vi "main0.1.vi"() -> ()   [LabVIEW 2025]
uses:
  STATES_MACHINE.ctl
  <vilib>/Utility/file.llb/Write Delimited Spreadsheet (DBL).vi
panel:
  out "array":dbl[][](array[numeric]) format="%#_5g"
  out "Enum":T1
  in  "Stop Generale":bool
  in  "Aggiungi caso":bool
  out "Outlet":dbl
  out "Secondary":dbl
  out "Primary":dbl
  out "Waveform Graph":dynamicdata(graph)
  in  "Altro test":bool
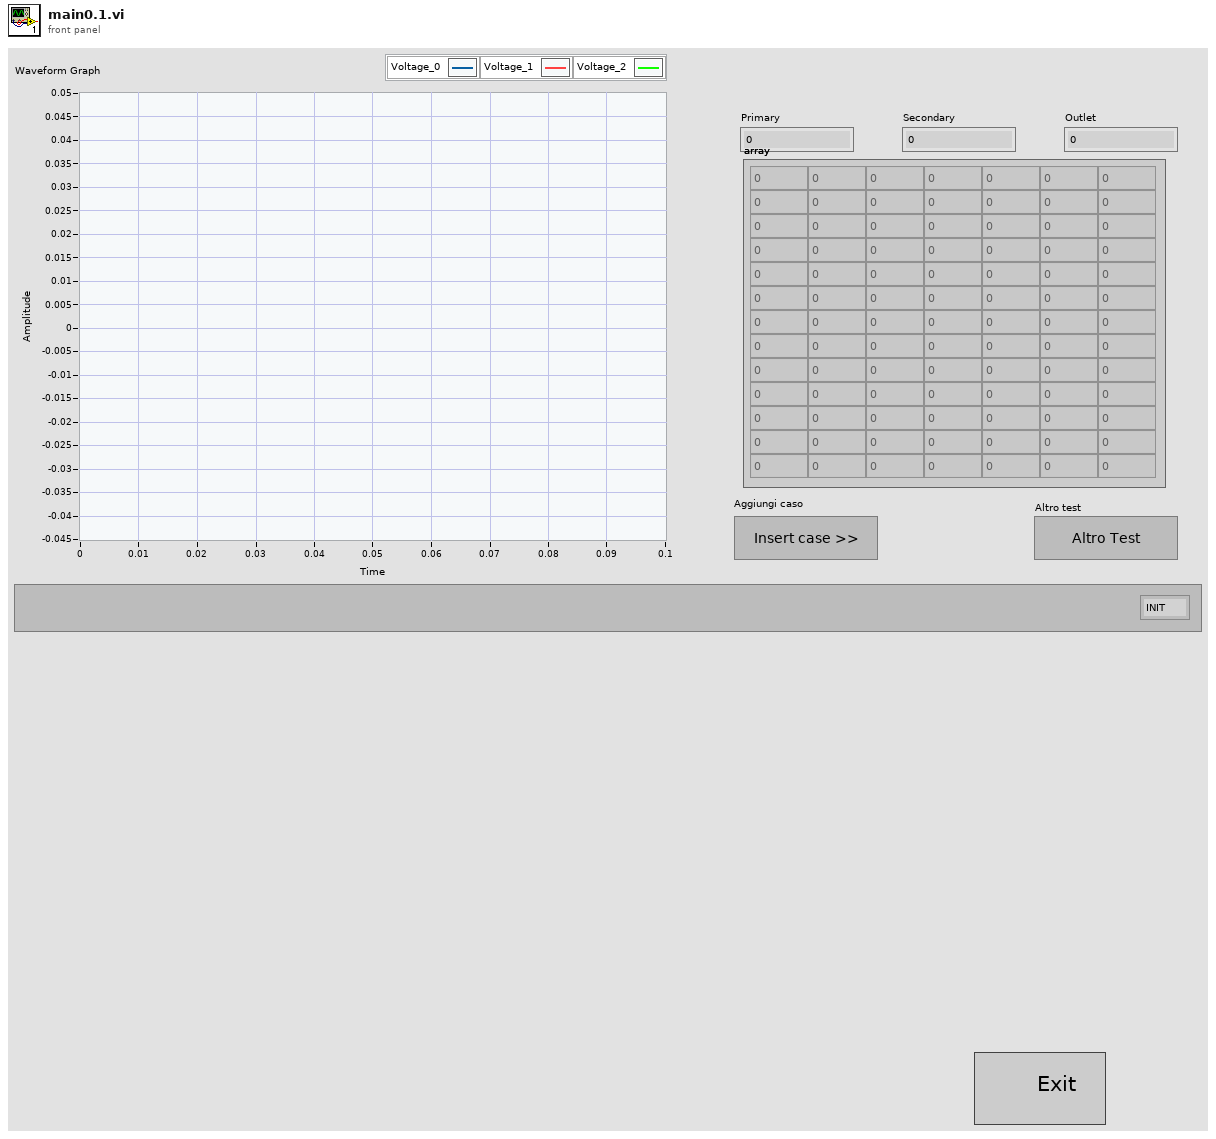
[diagram p1: front panel]
types:
  T1 = typedef "STATES_MACHINE.ctl" = enum16{"INIT", "TEST", "WRITE_RESULT", "CLOSE"}
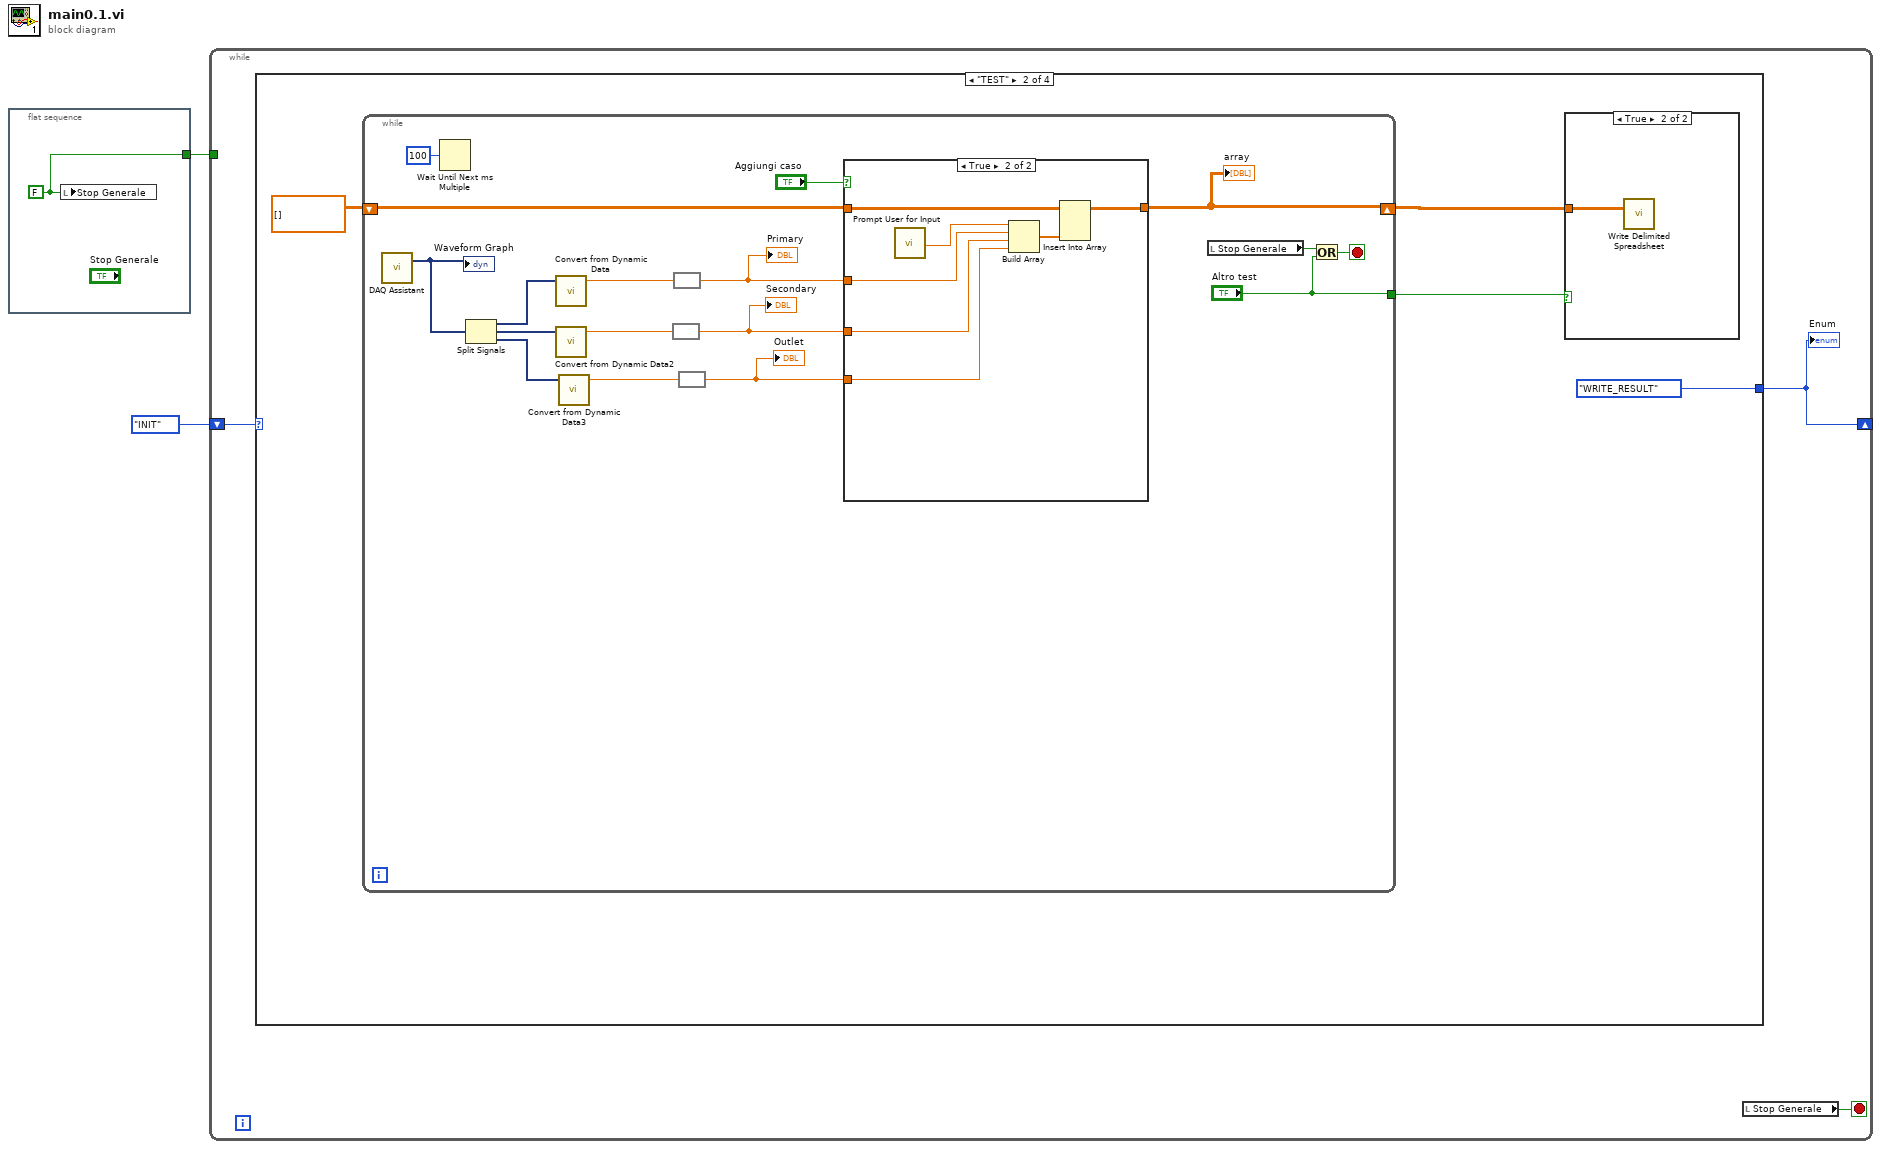
[diagram p0: block diagram]
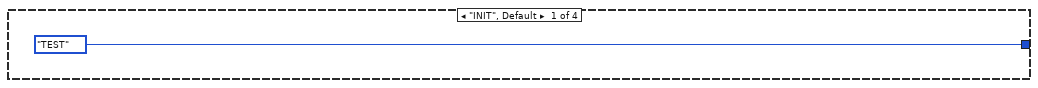
[diagram p2: hidden frame]
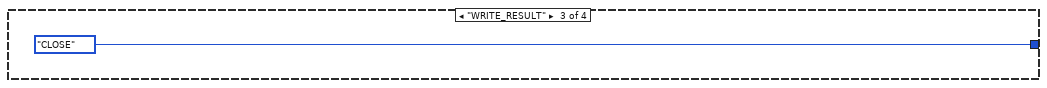
[diagram p5: hidden frame]
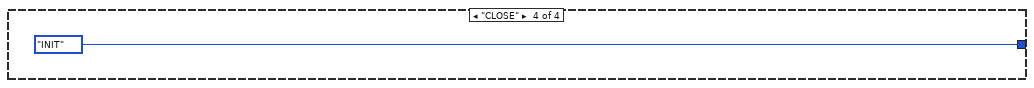
[diagram p6: hidden frame]
diagram:
  n1 = flat-sequence {
    tunnel: [w3] -> w1
    frame #0 {
      w3 = FALSE ("Stop Button 2")
      n2 = local write "Stop Generale"(w3) -> ()
    }
  }
  n3 = while {
    shift-right: [w5] -> _
    shift-left: STATES_MACHINE."INIT" ("Enum") -> [w6]
    tunnel: w1 -> [_]
    stop <- w4 stop-if-true
    n4 = case shown="\"TEST\"" w6 {
      tunnel: [STATES_MACHINE."TEST" ("Enum") STATES_MACHINE."WRITE_RESULT" ("Enum") STATES_MACHINE."CLOSE" ("Enum") STATES_MACHINE."INIT" ("Enum")] -> w5
      frame "INIT", Default {
      }
      frame "TEST" {
        n5 = while {
          shift-right: [w19] -> w9
          shift-left: dbl[][] [] ("array") -> [w20]
          tunnel: ["Altro test"] -> w8
          stop <- w18 stop-if-true
          n6 = call "DAQ Assistant"() -> ("data"=w25:dynamicdata)  [unwired: 17 in, 2 out]
          "Waveform Graph" <- w25
          n7 = Wait Until Next ms Multiple(millisecond multiple=u32 100) -> ()  [unwired: 1 out]
          n8 = Split Signals(w25) -> (w28:dynamicdata, w27:dynamicdata, w26:dynamicdata)  [unwired: 3 in]
          n9 = call "Convert from Dynamic Data"("Dynamic Data Type"=w28) -> ("Scalar"=w23:dbl)  [unwired: 3 in]
          n10 = call "Convert from Dynamic Data2"("Dynamic Data Type"=w27) -> ("Scalar"=w22:dbl)  [unwired: 3 in]
          n11 = call "Convert from Dynamic Data3"("Dynamic Data Type"=w26) -> ("Scalar"=w21:dbl)  [unwired: 3 in]
          n12 = expression code=""(w22) -> (w14:dbl)
          "Secondary" <- w14
          n13 = expression code=""(w23) -> (w15:dbl)
          "Primary" <- w15
          n14 = expression code=""(w21) -> (w13:dbl)
          "Outlet" <- w13
          n15 = case shown="True" "Aggiungi caso" {
            tunnel: w15 -> [_ w35]
            tunnel: w14 -> [_ w34]
            tunnel: w13 -> [_ w33]
            tunnel: w20 -> [w30 w37]
            tunnel: [w30 w36] -> w19
            frame False {
            }
            frame True {
              n16 = call "Prompt User for Input"() -> ("Current"=w31:dbl)  [unwired: 17 in, 2 out]
              n17 = Build Array(w31, w35, w34, w33) -> (w32:dbl[])
              n18 = Insert Into Array(array=w37, new element=w32) -> (w36:dbl[][])  [unwired: 2 in]
            }
          }
          "array" <- w19
          n19 = local read "Stop Generale"() -> (w17:bool)
          n20 = Or(x=w17, y="Altro test") -> (x .or. y?=w18:bool)
        }
        n21 = case shown="True" w8 {
          tunnel: w9 -> [_ w12]
          frame False {
          }
          frame True {
            n22 = call-poly <vilib>:"Write Delimited Spreadsheet.vi"("2D data"=w12) -> ()  [unwired: 13 in, 2 out]
          }
        }
      }
      frame "WRITE_RESULT" {
      }
      frame "CLOSE" {
      }
    }
    "Enum" <- w5
    n23 = local read "Stop Generale"() -> (w4:bool)
  }
